vi "jacktutorial.vi"() -> ()   [LabVIEW 2014]
panel:
  in  "Description":string
  out "Datafile 1":path
  out "XY Graph":cluster{"X":dbl[], "Y":dbl[]}[](graph)
  in  "f(x)":u16(ring) items=["sin(x)", "x^2", "x^3", "sqrt(x)", "f(x)=x"]
  out "y_array":dbl[](array[numeric])
  out "x_squared":dbl[](array[numeric])
  out "x_array":dbl[](array[numeric])
  out "x_steps":dbl
  in  "x_res":dbl
  in  "x_end":dbl
  in  "x_start":dbl
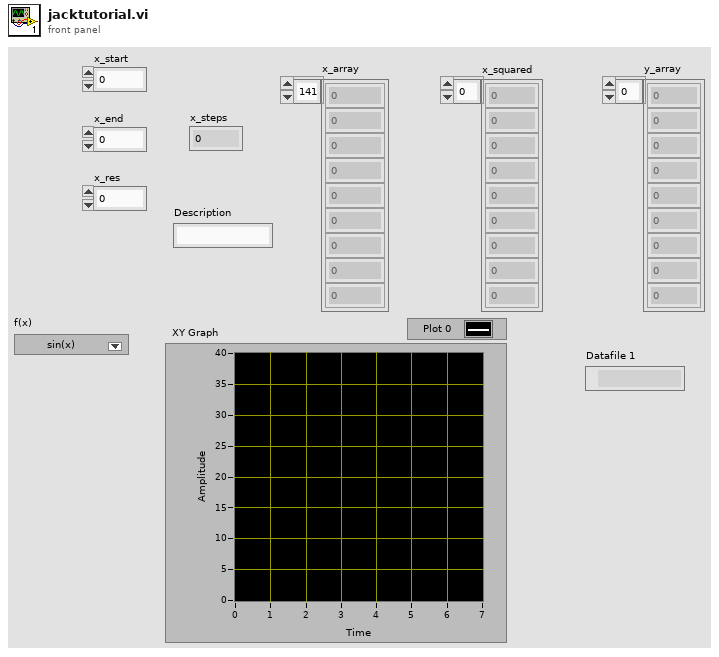
[diagram p1: front panel]
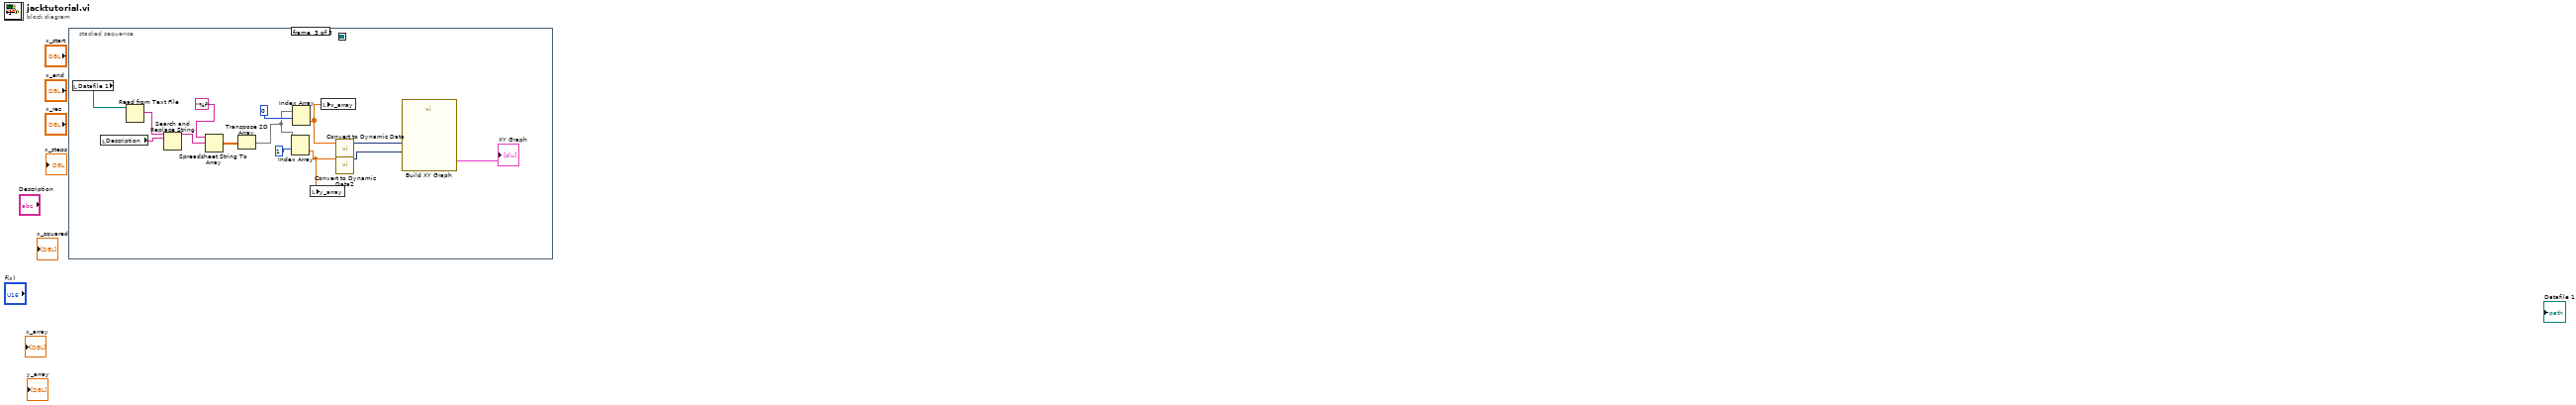
[diagram p0: block diagram]
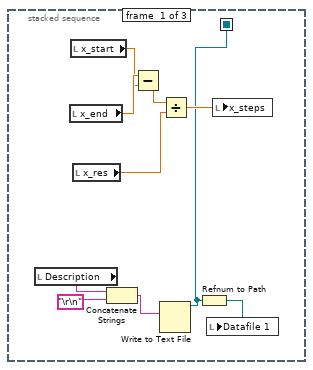
[diagram p2: hidden frame]
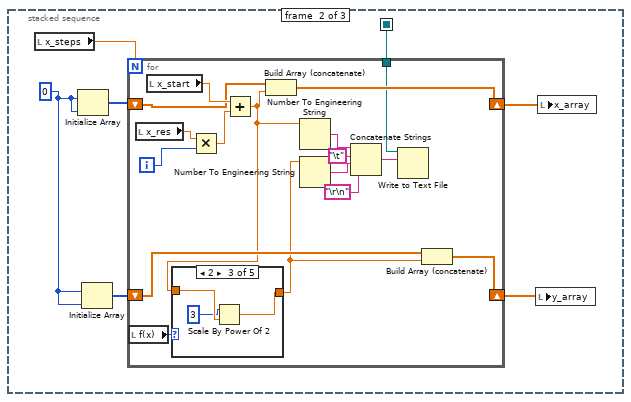
[diagram p3: hidden frame]
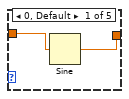
[diagram p4: hidden frame]
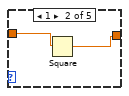
[diagram p5: hidden frame]
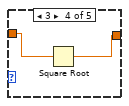
[diagram p6: hidden frame]
diagram:
  n1 = stacked-sequence {
    seq-local: [w1 _ _] -> [_ w11 _]
    frame #0 {
      n2 = local read "Description"() -> (w4:string)
      n3 = local read "x_end"() -> (w10:dbl)
      n4 = local read "x_start"() -> (w9:dbl)
      n5 = local read "x_res"() -> (w7:dbl)
      n6 = Concatenate Strings(w4, "\r\n") -> (w3:string)
      n7 = Subtract(x=w10, y=w9) -> (x-y=w8:dbl)
      n8 = Write to Text File(text=w3) -> (refnum out=w1:refnum<file>)  [unwired: 3 in, 2 out]
      n9 = Divide(x=w8, y=w7) -> (x/y=w6:dbl)
      n10 = Refnum to Path(1:w1) -> (0:w2:path)
      n11 = local write "Datafile 1"(w2) -> ()
      n12 = local write "x_steps"(w6) -> ()
    }
    frame #1 {
      w13 = 0
      n13 = local read "x_steps"() -> (w17:dbl)
      n14 = Initialize Array(w13, w13) -> (w16:i32[])
      n15 = Initialize Array(w13, w13) -> (w14:i32[])
      n16 = for {
        N: w17 -> [_]
        shift-right: [w29] -> w15
        shift-left: w16 -> [w30]
        shift-right: [w28] -> w12
        shift-left: w14 -> [w27]
        tunnel: w11 -> [w19]
        i -> [w33]
        n17 = local read "f(x)"() -> (w18:u16)
        n18 = local read "x_res"() -> (w34:dbl)
        n19 = local read "x_start"() -> (w31:dbl)
        n20 = Multiply(x=w34, y=w33) -> (x*y=w32:dbl)
        n21 = Add(x=w31, y=w32) -> (x+y=w26:dbl)
        n22 = case shown="2" w18 {
          tunnel: w26 -> [w36 w38 w41 w43 w44]
          tunnel: [w35 w37 w40 w42 w44] -> w25
          frame 0, Default {
            n23 = Sine(x=w36) -> (sin(x)=w35:dbl)
          }
          frame 1 {
            n24 = Square(x=w38) -> (x^2=w37:dbl)
          }
          frame 2 {
            n25 = Scale By Power Of 2(n=3, x=w41) -> (x*2^n=w40:dbl)
          }
          frame 3 {
            n26 = Square Root(x=w43) -> (sqrt(x)=w42:dbl)
          }
          frame 4 {
          }
        }
        n27 = Build Array (concatenate)(w30, w26) -> (w29:dbl[])
        n28 = Number To Engineering String(4:w26) -> (0:w24:string)  [unwired: 3 in]
        n29 = Number To Engineering String(4:w25) -> (0:w23:string)  [unwired: 3 in]
        n30 = Concatenate Strings(w24, "\t", w23, "\r\n") -> (w20:string)
        n31 = Write to Text File(file (use dialog)=w19, text=w20) -> ()  [unwired: 2 in, 3 out]
        n32 = Build Array (concatenate)(w27, w25) -> (w28:dbl[])
      }
      n33 = local write "y_array"(w12) -> ()
      n34 = local write "x_array"(w15) -> ()
    }
    frame #2 {
      n35 = local read "Datafile 1"() -> (w45:path)
      n36 = local read "Description"() -> (w52:string)
      n37 = Read from Text File(file (use dialog)=w45) -> (text=w53:string)  [unwired: 3 in, 3 out]
      n38 = Search and Replace String(input string=w53, search string=w52) -> (result string=w51:string)  [unwired: 6 in, 3 out]
      n39 = Spreadsheet String To Array(format string="%f", spreadsheet string=w51) -> (array=w50:dbl[][])  [unwired: 2 in]
      n40 = Transpose 2D Array(2D array=w50) -> (transposed array=w49:dbl[][])
      n41 = Index Array(array=w49, index (row)=1) -> (element=w46:dbl[])  [unwired: 1 in]
      n42 = Index Array(array=w49, index (row)=0) -> (element=w47:dbl[])  [unwired: 1 in]
      n43 = local write "y_array"(w46) -> ()
      n44 = local write "x_array"(w47) -> ()
      n45 = call "Convert to Dynamic Data"("Array"=w47) -> ("Dynamic Data Type"=w58:dynamicdata)  [unwired: 3 in]
      n46 = call "Convert to Dynamic Data2"("Array"=w46) -> ("Dynamic Data Type"=w57:dynamicdata)  [unwired: 3 in]
      n47 = call "Build XY Graph"("Y Input"=w57, "X Input"=w58) -> ("XY Graph"=→"XY Graph":cluster{"X":dbl[], "Y":dbl[]}[])  [unwired: 8 in, 1 out]
    }
  }
